vi "Unflatten.vi"(8 "error in":errorcluster, 10 "Buffer":u8[](array[numeric]) format="%.0x") -> (0 "error out":errorcluster, 2 "Data":T1)   [LabVIEW 2020, in "CmdAnalog.lvlib"]
uses:
  CmdAnalog.lvlib
  Data.ctl
  lv-protoc/LV-Proto/Wire Decode Varint I32.vi
  lv-protoc/LV-Proto/Extract Varint Bytes.vi
  lv-protoc/LV-Proto/LV-Proto.lvlib
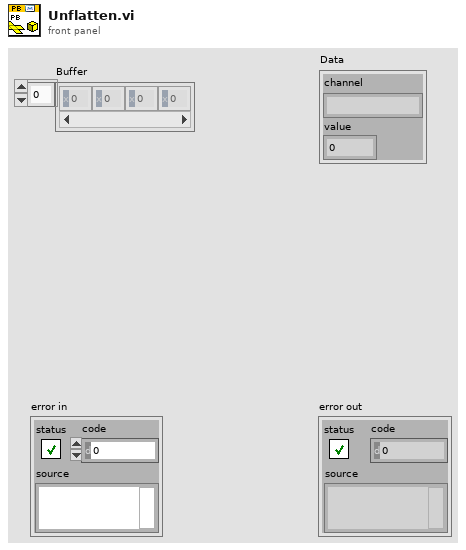
[diagram p1: front panel]
types:
  T1 = typedef "CmdAnalog.lvlib/Data.ctl" = cluster{"channel":string, "value":dbl}
  T2 = typedef "LV-Proto.lvlib/Wire Type.ctl" = enum8{"VARINT", "I64", "LEN", "SGROUP (Deprecated)", "EGROUP (Deprecated)", "I32"}
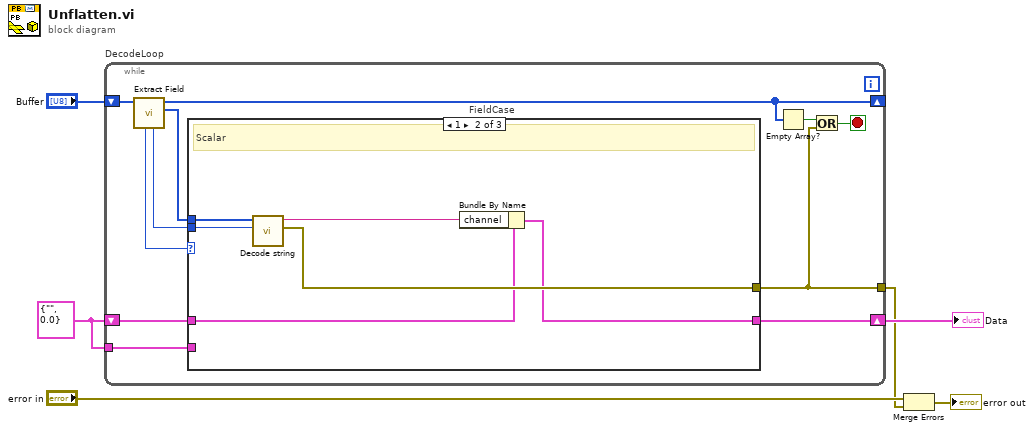
[diagram p0: block diagram]
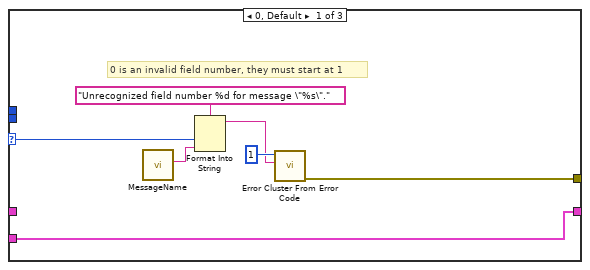
[diagram p2: hidden frame]
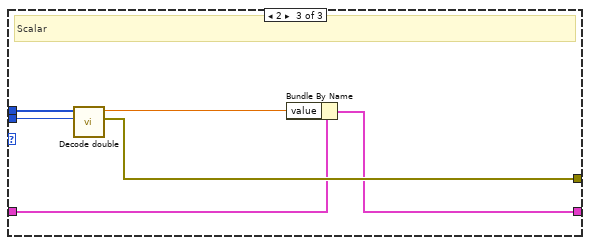
[diagram p3: hidden frame]
diagram:
  w4 = T1 {"channel"="", "value"=0.0} ("Data")
  n1 = while "DecodeLoop" {
    shift-right: [w16] -> _
    shift-left: "Buffer" -> [w17]
    shift-right: [w9] -> w5
    shift-left: w4 -> [w15]
    tunnel: [w8] -> w2
    tunnel: w4 -> [w7]
    stop <- w11 stop-if-true
    n2 = call "Extract Field.vi"("Buffer in"=w17) -> ("Field Data"=w10:u8[], "Buffer"=w16:u8[], "Wire Type"=w13:T2, "Field Number"=w14:i32)  [unwired: 7 in]
    n3 = case "FieldCase" shown="1" w14 {
      selector: w14 -> [w23 _ _]
      tunnel: w15 -> [_ w26 w32]
      tunnel: w13 -> [_ w28 w34]
      tunnel: w10 -> [_ w29 w35]
      tunnel: [w19 w25 w31] -> w9
      tunnel: [w20 w30 w36] -> w8
      tunnel: w7 -> [w19 _ _]
      frame 0, Default {
        # "0 is an invalid field number, they must start at 1"
        n4 = call "MessageName.vi"() -> ("MessageName"=w18:string)  [unwired: 11 in]
        n5 = Format Into String(format string="Unrecognized field number %d for message \"%s\".", w23, w18) -> (resulting string=w21:string)  [unwired: 2 in, 1 out]
        n6 = call <vilib>:"Error Cluster From Error Code.vi"("error message (\"\")"=w21, "error code (0)"=1) -> ("error out"=w20:errorcluster)  [unwired: 7 in]
      }
      frame 1 {
        # "Scalar"
        n7 = call "Decode string.vi"("Wire Type"=w28, "Data"=w29) -> ("error out"=w30:errorcluster, "string"=w27:string)  [unwired: 8 in]
        n8 = Bundle By Name(cluster=w26, "channel"=w27) -> (w25:T1)
      }
      frame 2 {
        # "Scalar"
        n9 = call "Decode double.vi"("Wire Type"=w34, "Data"=w35) -> ("error out"=w36:errorcluster, "double"=w33:dbl)  [unwired: 8 in]
        n10 = Bundle By Name(cluster=w32, "value"=w33) -> (w31:T1)
      }
    }
    n11 = Empty Array?(array=w16) -> (empty?=w12:bool)
    n12 = Or(x=w12, y=w8) -> (x .or. y?=w11:bool)
  }
  "Data" <- w5
  n13 = Merge Errors("error in", w2) -> (→"error out":errorcluster)
